vi "MotionVI.vi"(8 "Error In":errorcluster, 11 "AirSAS Controls in":T1 {"Waveform"."LFM Parameters"."Window %" format="%.2g"; "Waveform"."LFM Parameters"."Out. Amplitude (Vpk)" format="%0.2f"; "Waveform"."LFM Parameters"."Fstop (Hz)" format="%^.3e"; "Waveform"."LFM Parameters"."Fstart (Hz)" format="%^.3e"; "Waveform"."LFM Parameters"."Duration" format="%.3f"}) -> (0 "Error out":errorcluster, 3 "output cluster":T1={"Receive Duration"=0.0, "I/O"={"DAQmx Device"="Dev1", "AO Range"=0.0, "AI Range"=0.0, "DAQ Group Delay"=0.0, "Fs"=0.0}, "Hardware"={"Centerpos"=[0.0, 0.0, 0.0], "TXpos"=[0.0, 0.0, 0.0], "RX1pos"=[0.0, 0.0, 0.0], "RX2pos"=[0.0, 0.0, 0.0], "Angle"=0.0, "Height"=0.0}, "Waveform"={"LFM Parameters"={"Duration"=1.0, "Fstart (Hz)"=1000.0, "Fstop (Hz)"=10000.0, "Out. Amplitude (Vpk)"=1.0, "Window %"=10.0}, "Transmit Waveform"={"t0"=timestamp(0 s since 1904-01-01), "dt"=1.0, "Y"=[]}}, "LINX Resource"={"IO"=enum."Remote", "Interface"=enum."Serial", "LINX Device Config"={"Interface"=enum."Serial", "COM Port"="COM13", "TCP Configuration"={"IP Address"="", "Port"=0}, "Device Family"=1, "Device ID"=1, "Device Name"="myRIO-1900", "TCP Ref"=refnum, "Channels"={"DI"=[0, 1, 2, 3, 4, 5, 6, 7, 8, 9, 10, 11, 12, 13, 14, 15, 16, 17, 18, 19, 20, 21, 22, 23, 24, 25, 26, 27, 28, 29, 30, 31, 32, 33, 34, 35, 36, 37, 38, 39, 40, 41, 42, 43, 44, 45, 46], "DO"=[0, 1, 2, 3, 4, 5, 6, 7, 8, 9, 10, 11, 12, 13, 14, 15, 16, 17, 18, 19, 20, 21, 22, 23, 24, 25, 26, 27, 28, 29, 30, 31, 32, 33, 34, 35, 36, 37, 38, 39, 40, 41, 42, 43, 44, 45, 46], "AI"=[0, 1, 2, 3, 4, 5, 6, 7, 8, 9, 10, 11], "AO"=[], "PWM"=[3, 5, 6, 9, 10], "QE"=[], "UART"=[0, 1], "I2C 2"=[0], "SPI"=[0], "CAN"=[], "Servo"=[], "AI Ref (V)"=0.0, "AI Resolution (Bits)"=0, "AO Ref (V)"=0.0, "AO Resolution (Bits)"=0}}}, "Port"=3000.0} {"Waveform"."LFM Parameters"."Window %" format="%.2g"; "Waveform"."LFM Parameters"."Out. Amplitude (Vpk)" format="%0.2f"; "Waveform"."LFM Parameters"."Fstop (Hz)" format="%^.3e"; "Waveform"."LFM Parameters"."Fstart (Hz)" format="%^.3e"; "Waveform"."LFM Parameters"."Duration" format="%.3f"})   [LabVIEW 2018]
doc: "Use this VI to request control the motion of the turntable. The front panel of the VI, shown below, allows the user to control both the rotation and vertical motion of the table. The controls include whether or not the motors are enabled, the frequency of the motor, how much distance should be covered, and direction, along with buttons to start and stop the motion. You can also specify the serial port the Arduino is plugged into."
uses:
  N:/SRDD-Student/Ng/fromTom/Air SAS Data Acquisition/controls/Air SAS Controls.ctl
  <vilib>/MakerHub/LINX/Private/Type Defs/LINX Ref.ctl
  <vilib>/MakerHub/LINX/Private/Type Defs/Platform.ctl
  <vilib>/MakerHub/LINX/Private/Type Defs/Interface.ctl
  <vilib>/MakerHub/LINX/Private/Device/Type Defs/LINX Device Config.ctl
  <vilib>/MakerHub/LINX/Private/Device/Type Defs/TCP Config.ctl
  <vilib>/MakerHub/LINX/Private/Device/Type Defs/Channels.ctl
  <vilib>/Utility/error.llb/DialogType.ctl
  <vilib>/MakerHub/LINX/Public/Peripherals/Digital/Digital Write 1 Chan.vi
  <vilib>/MakerHub/LINX/Public/Peripherals/Digital/Digital Write N Chans.vi
  <vilib>/MakerHub/LINX/Private/Local IO/LinxDigitalWrite.vi
  <vilib>/MakerHub/LINX/Public/Utilities/Check Channel.vi
  <vilib>/MakerHub/LINX/Private/Utilties/Generate Error.vi
  <vilib>/MakerHub/LINX/LMH-LINX.lvlib
  <vilib>/MakerHub/LINX/Private/Device/Device.lvlib
panel:
  in  "Move":bool
  in  "ccw/cw":bool
  in  "up/down":bool
  out "?":string
  in  "Frequency (Hz)":u32=650 format="%.2f"
  in  "Millimeters":dbl=1.0
  in  "Enable 2":bool
  in  "stop 2":bool
  out "?":string
  in  "Rotate Frequency (Hz)":u32=1000 format="%.2f"
  in  "Degrees":dbl=1.0
  in  "Rotate":bool
  in  "Enable":bool
  in  "stop":bool
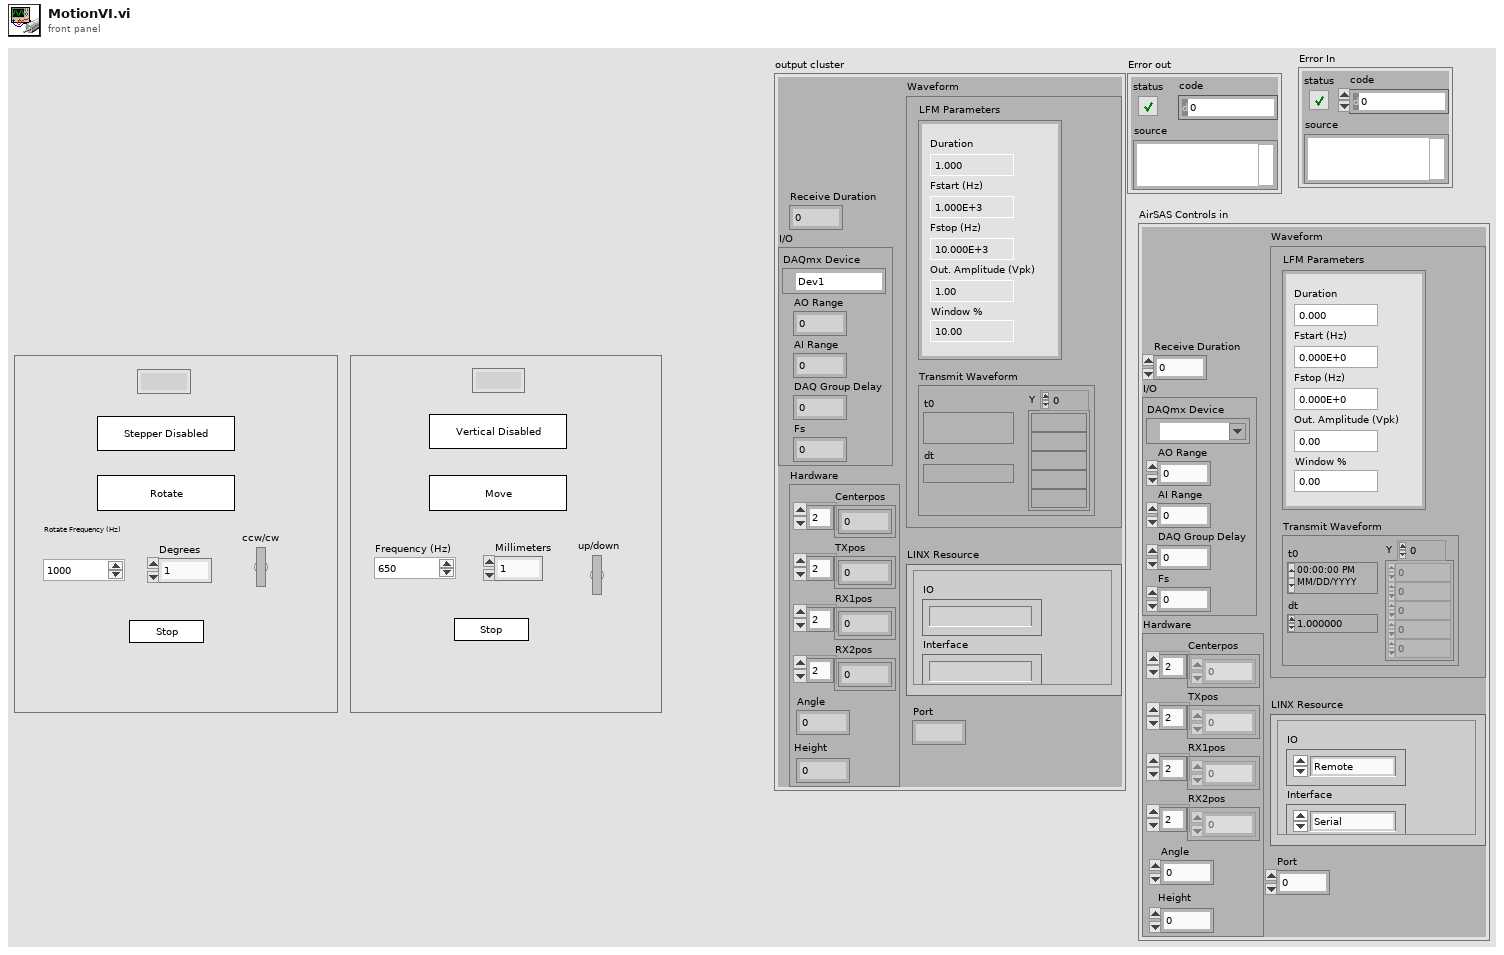
[diagram p1: front panel]
types:
  T1 = typedef "Air SAS Controls.ctl" = cluster{"Receive Duration":dbl, "I/O":cluster{"DAQmx Device":tag, "AO Range":dbl, "AI Range":dbl, "DAQ Group Delay":dbl, "Fs":dbl}, "Hardware":cluster{"Centerpos":dbl[], "TXpos":dbl[], "RX1pos":dbl[], "RX2pos":dbl[], "Angle":dbl, "Height":dbl}, "Waveform":cluster{"LFM Parameters":cluster{"Duration":dbl, "Fstart (Hz)":dbl, "Fstop (Hz)":dbl, "Out. Amplitude (Vpk)":dbl, "Window %":dbl}, "Transmit Waveform":waveform(dbl)}, "LINX Resource":T2, "Port":dbl}
  T2 = typedef "LMH-LINX.lvlib/LINX Ref.ctl" = cluster{"IO":T3, "Interface":T4, "LINX Device Config":T5}
  T3 = typedef "LMH-LINX.lvlib/Platform.ctl" = enum16{"Remote", "Local"}
  T4 = typedef "LMH-LINX.lvlib/Interface.ctl" = enum16{"Serial", "TCP"}
  T5 = typedef "LMH-LINX.lvlib/Device.lvlib/LINX Device Config.ctl" = cluster{"Interface":T4, "COM Port":refnum<visa-resource-name>, "TCP Configuration":T6, "Device Family":u8, "Device ID":u8, "Device Name":string, "TCP Ref":refnum<k5>, "Channels":T7}
  T6 = typedef "LMH-LINX.lvlib/Device.lvlib/TCP Config.ctl" = cluster{"IP Address":string, "Port":u16}
  T7 = typedef "LMH-LINX.lvlib/Channels.ctl" = cluster{"DI":u8[], "DO":u8[], "AI":u8[], "AO":u8[], "PWM":u8[], "QE":u8[], "UART":u8[], "I2C 2":u8[], "SPI":u8[], "CAN":u8[], "Servo":u8[], "AI Ref (V)":dbl, "AI Resolution (Bits)":u8, "AO Ref (V)":dbl, "AO Resolution (Bits)":u8}
  T8 = typedef "DialogType.ctl" = u16
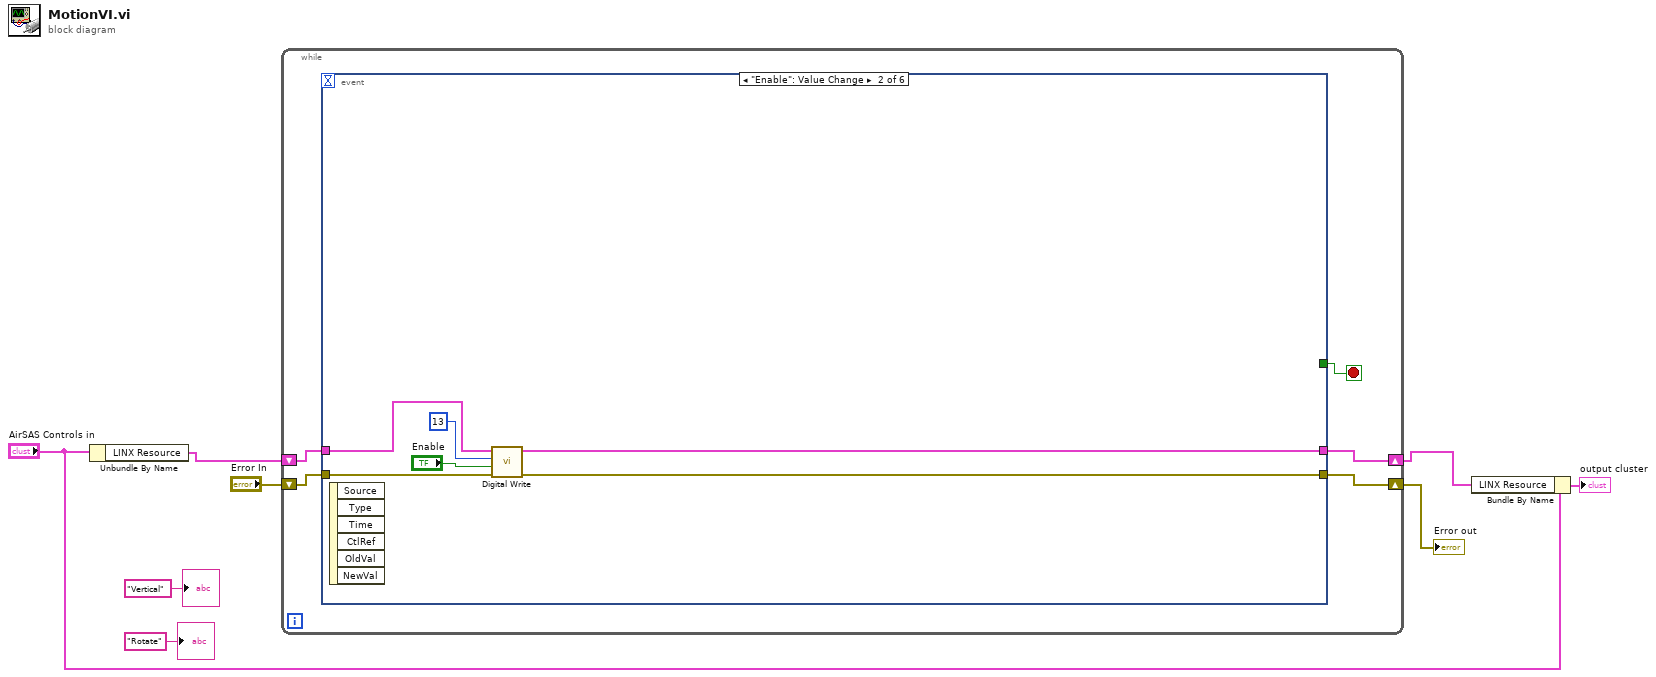
[diagram p0: block diagram]
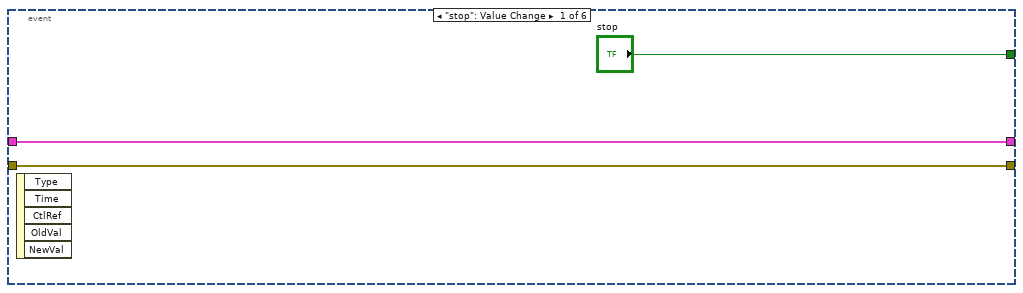
[diagram p2: hidden frame]
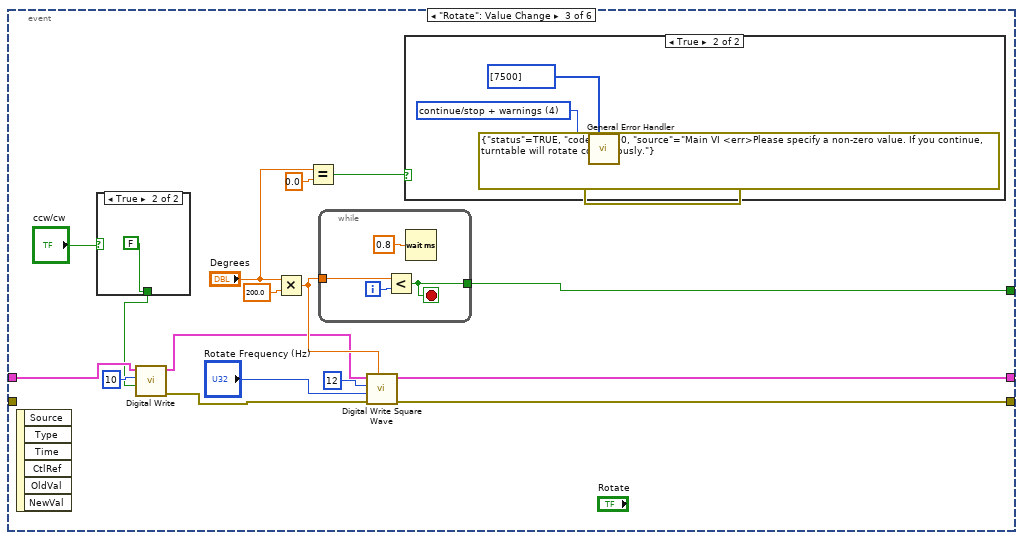
[diagram p3: hidden frame]
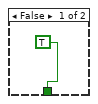
[diagram p4: hidden frame]
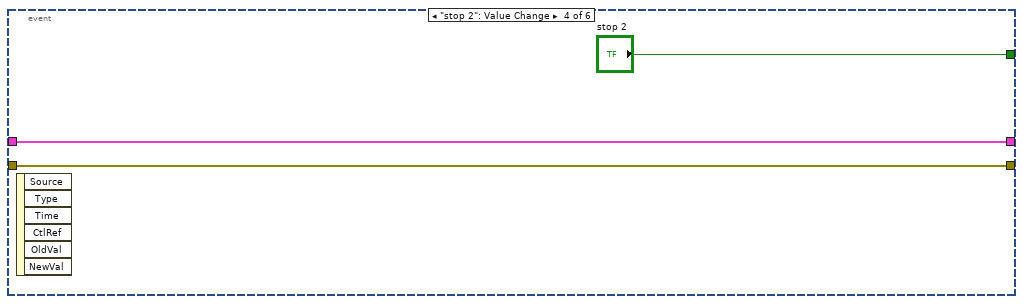
[diagram p6: hidden frame]
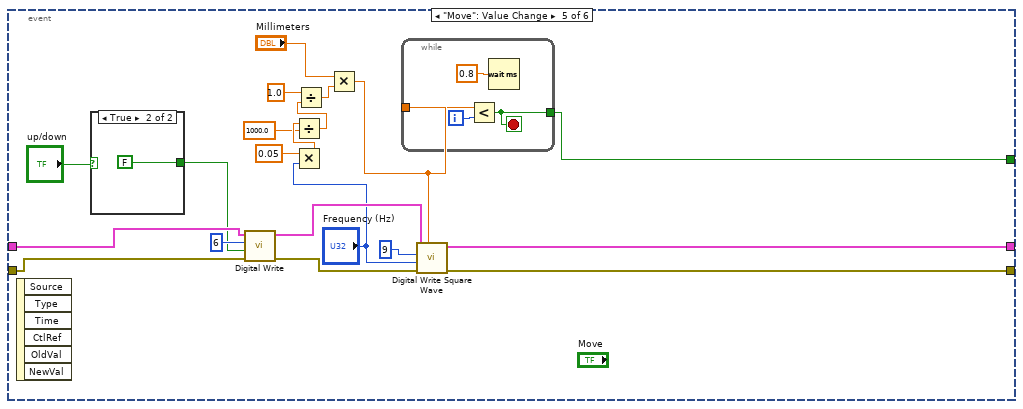
[diagram p7: hidden frame]
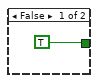
[diagram p8: hidden frame]
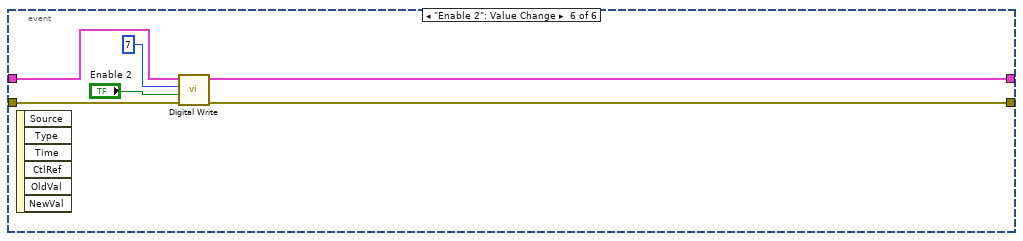
[diagram p9: hidden frame]
diagram:
  n1 = Unbundle By Name("AirSAS Controls in") -> ("LINX Resource"=w6:T2)
  n2 = while {
    shift-right: [w11] -> w1
    shift-left: "Error In" -> [w12]
    shift-right: [w10] -> w5
    shift-left: w6 -> [w13]
    stop <- w9 stop-if-true
    n3 = event shown="[1] \"Enable\": Value Change" {
      selector: _ -> [_ _ _ _ _ _]
      dyn-events: _ -> [_ _ _ _ _ _]
      timeout: _ -> [_ _ _ _ _ _]
      tunnel: ["stop" _ w30 "stop 2" w67 _] -> w9
      tunnel: w13 -> [w15 w22 w26 w49 w63 w81]
      tunnel: w12 -> [w14 w21 _ w48 w62 w80]
      tunnel: [w14 w19 w38 w48 w68 w78] -> w11
      tunnel: [w15 w18 w37 w49 w69 w79] -> w10
      event "stop": Value Change {
        n4 = event-data() -> ()  [unwired: 1 in, 5 out]
      }
      event "Enable": Value Change {
        n5 = event-data() -> ()  [unwired: 1 in, 6 out]
        n6 = call-poly <vilib>:"Digital Write.vi"("Error In"=w21, "Output Value"="Enable", "DO Channel"=u8 13 ("EN Channel"), "LINX Resource"=w22) -> ("Error Out"=w19:errorcluster, "LINX Resource"=w18:T2)  [unwired: 6 in]
      }
      event "Rotate": Value Change {
        n7 = event-data() -> ()  [unwired: 1 in, 6 out]
        n8 = case shown="True" "ccw/cw" {
          tunnel: [TRUE FALSE] -> w25
          frame False {
          }
          frame True {
          }
        }
        n9 = call-poly <vilib>:"Digital Write.vi"("Output Value"=w25, "DO Channel"=u8 10 ("DIR channel"), "LINX Resource"=w26) -> ("Error Out"=w23:errorcluster, "LINX Resource"=w24:T2)  [unwired: 7 in]
        n10 = Multiply(x="Degrees", y=200.0) -> (x*y=w29:dbl)
        n11 = Equal?(x="Degrees", y=0.0) -> (x = y?=w32:bool)
        n12 = while {
          tunnel: w29 -> [w44]
          tunnel: [w41] -> w30
          i -> [w43]
          stop <- w41 stop-if-true
          n13 = Less?(x=w44, y=w43) -> (x < y?=w41:bool)
          n14 = Wait (ms)(milliseconds to wait=0.8) -> ()  [unwired: 1 out]
        }
        n15 = call <vilib>:"Digital Write Square Wave.vi"("Duration (ms)"=w29, "Error In"=w23, "Frequency (Hz)"="Rotate Frequency (Hz)", "Channel"=u8 12 ("Digital Output Channel"), "LINX Resource"=w24) -> ("Error Out"=w38:errorcluster, "LINX Resource"=w37:T2)  [unwired: 5 in]
        n16 = case shown="True" w32 {
          frame False {
          }
          frame True {
            w46 = T8 4 items=["no dialog", "OK message", "continue or stop message", "OK message + warnings", "continue/stop + warnings"] ("type of dialog (OK msg:1)")
            n17 = call <vilib>:"General Error Handler.vi"("[user-defined codes]"=i32[] [7500], "type of dialog (OK msg:1)"=w46, "error in (no error)"=errorcluster {"status"=TRUE, "code"=7500, "source"="Main VI <err>Please specify a non-zero value. If you continue, turntable will rotate continuously."}) -> ()  [unwired: 8 in, 5 out]
          }
        }
      }
      event "stop 2": Value Change {
        n18 = event-data() -> ()  [unwired: 1 in, 6 out]
      }
      event "Move": Value Change {
        n19 = event-data() -> ()  [unwired: 1 in, 6 out]
        n20 = case shown="True" "up/down" {
          tunnel: [TRUE FALSE] -> w60
          frame False {
          }
          frame True {
          }
        }
        n21 = call-poly <vilib>:"Digital Write.vi"("Error In"=w62, "Output Value"=w60, "DO Channel"=u8 6 ("DIR channel"), "LINX Resource"=w63) -> ("Error Out"=w61:errorcluster, "LINX Resource"=w64:T2)  [unwired: 6 in]
        n22 = Multiply(x=0.05 ("y"), y="Frequency (Hz)") -> (x*y=w55:dbl)
        n23 = Divide(x=w55, y=1000.0 ("x")) -> (x/y=w52:dbl)
        n24 = Divide(x=1.0, y=w52) -> (x/y=w51:dbl)
        n25 = Multiply(x="Millimeters", y=w51) -> (x*y=w58:dbl)
        n26 = while {
          tunnel: w58 -> [w76]
          tunnel: [w73] -> w67
          i -> [w75]
          stop <- w73 stop-if-true
          n27 = Less?(x=w76, y=w75) -> (x < y?=w73:bool)
          n28 = Wait (ms)(milliseconds to wait=0.8) -> ()  [unwired: 1 out]
        }
        n29 = call <vilib>:"Digital Write Square Wave.vi"("Duration (ms)"=w58, "Error In"=w61, "Frequency (Hz)"="Frequency (Hz)", "Channel"=u8 9 ("Digital Output Channel"), "LINX Resource"=w64) -> ("Error Out"=w68:errorcluster, "LINX Resource"=w69:T2)  [unwired: 5 in]
      }
      event "Enable 2": Value Change {
        n30 = event-data() -> ()  [unwired: 1 in, 6 out]
        n31 = call-poly <vilib>:"Digital Write.vi"("Error In"=w80, "Output Value"="Enable 2", "DO Channel"=u8 7 ("EN Channel"), "LINX Resource"=w81) -> ("Error Out"=w78:errorcluster, "LINX Resource"=w79:T2)  [unwired: 6 in]
      }
    }
  }
  "Error out" <- w1
  n32 = Bundle By Name(cluster="AirSAS Controls in", "LINX Resource"=w5) -> (→"output cluster":T1)
  "?" <- "Vertical"
  "?" <- "Rotate"
